vi "Make a Token.vi"() -> ()   [LabVIEW 2021]
uses:
  <vilib>/Utility/sysdir.llb/System Directory Type.ctl
  <vilib>/LabVIEW Icon API/API_User Layer Data.ctl
  <vilib>/Utility/miscctls.llb/LVPoint32TypeDef.ctl
  <vilib>/picture/picture.llb/imagedata.ctl
  <vilib>/Utility/miscctls.llb/LVPositionTypeDef.ctl
  <vilib>/LabVIEW Icon API/lv_icon/Classes/Icon/Icon.lvclass
  Material-Scheme/Material-Scheme.lvclass
  <vilib>/LabVIEW Icon API/LabVIEW Icon API.lvlib
panel:
  in  "New Color":u32(colorbox)=5263440
  in  "VI with Control":path=path "C:/Development/Open Source/tsc-material-theme/other-buttons/source/palette/token--image.vi"
  out "appended path":path[](array[path])
  in  "File Path":path[](array[path])
  out "error out":errorcluster
  in  "error in":errorcluster
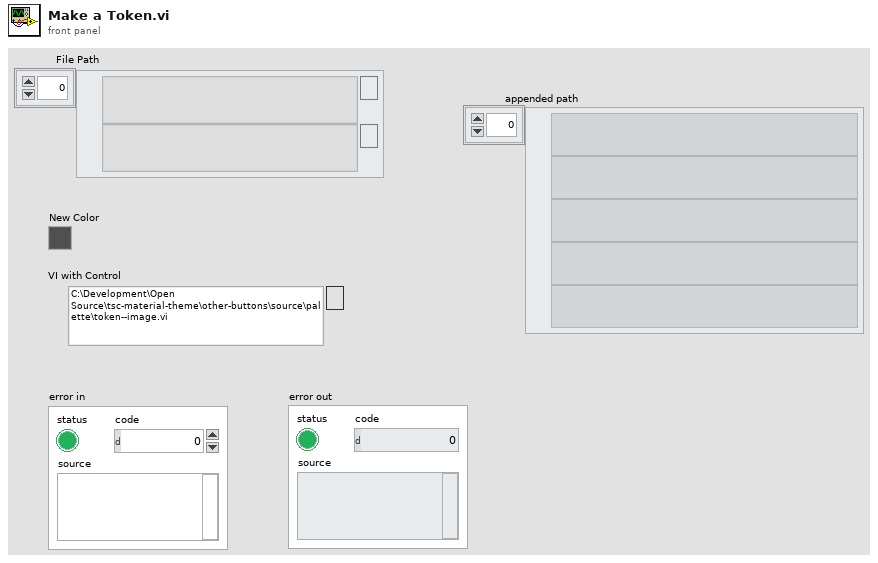
[diagram p1: front panel]
types:
  T1 = typedef "System Directory Type.ctl" = i32
  T2 = typedef "LVPoint32TypeDef.ctl" = cluster{"Horizontal":i32, "Vertical":i32}
  T3 = typedef "LabVIEW Icon API.lvlib/API_User Layer Data.ctl" = cluster{"Layer name":string, "Origin":T2, "Icon image data":T4}
  T4 = typedef "imagedata.ctl" = cluster{"image type":i32, "image depth":i32, "image":u8[], "mask":u8[], "colors":u32[], "Rectangle":cluster{"left":i16, "top":i16, "right":i16, "bottom":i16}}
  T5 = typedef "LVPositionTypeDef.ctl" = cluster{"Left":i32, "Top":i32}
  T6 = enum32{"invalid VI type", "Standard VI", "Control VI", "Global VI", "Polymorphic VI", "Configuration VI", "SubSystem", "Facade VI", "Method VI", "Statechart Diagram VI"}
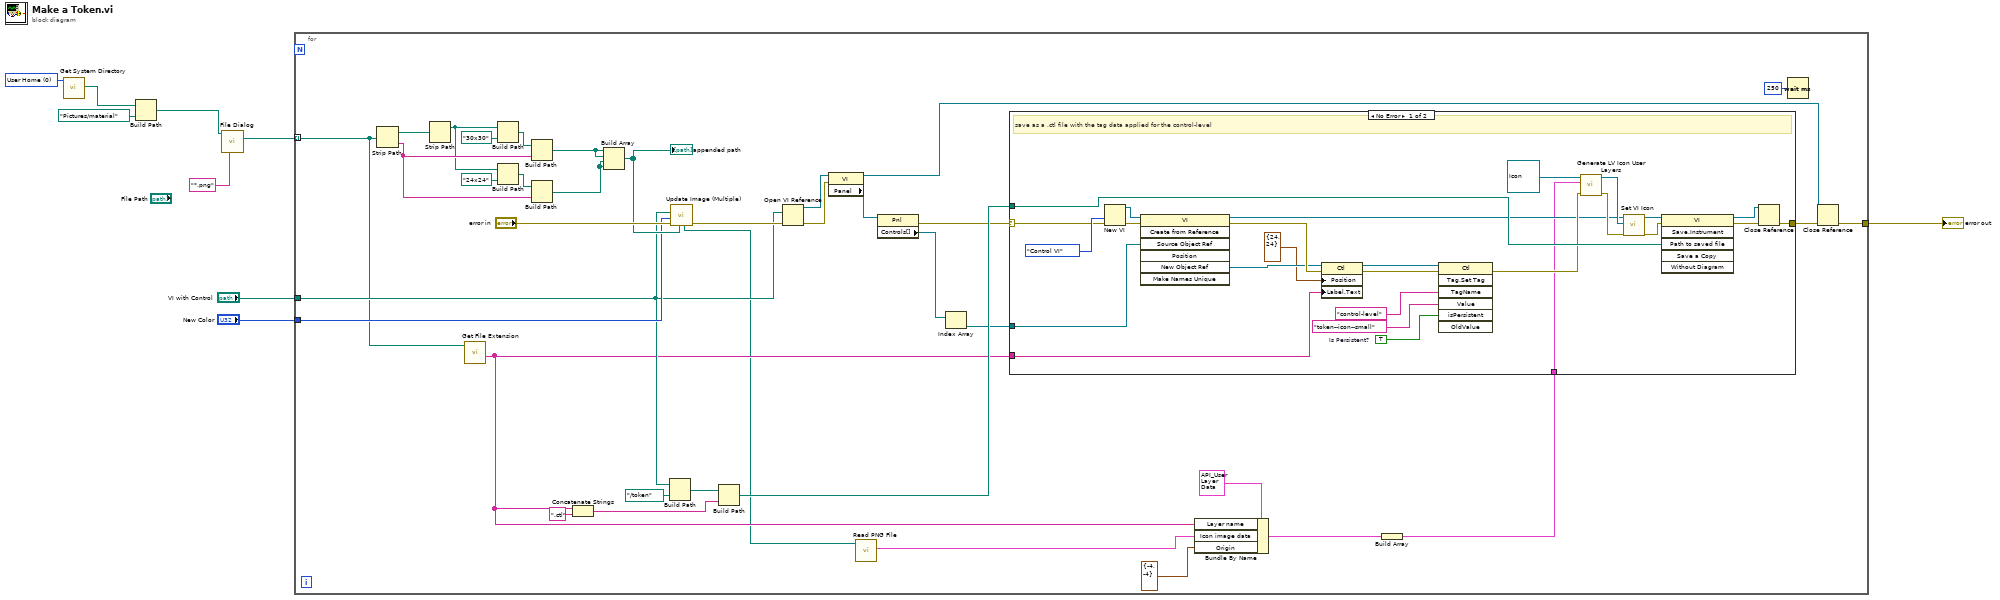
[diagram p0: block diagram]
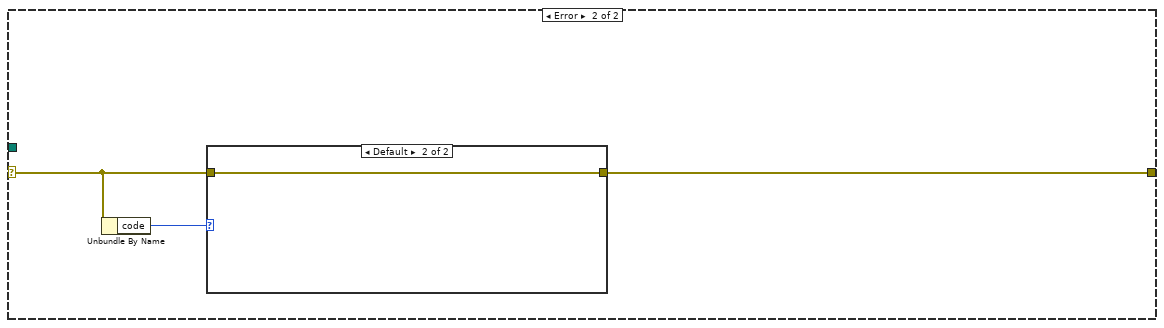
[diagram p2: hidden frame]
diagram:
  w4 = T1 0 items=["User Home"=0, "User Desktop"=1, "User Documents"=2, "User Application Data"=3, "User Preferences"=4, "User Temporary"=5, "Public Documents"=6, "Public Application Data"=7, "Public Preferences"=8, "Public Cache"=13, "System Core Libraries"=9, "System Installed Libraries"=10, "Application Files"=11, "Boot Volume Root"=12] ("system directory type")
  n1 = call <vilib>:"Get System Directory.vi"("system directory type"=w4) -> ("system directory"=w3:path)  [unwired: 10 in]
  n2 = Build Path(base path=w3, name or relative path=path "Pictures/material") -> (appended path=w1:path)
  n3 = call "File Dialog"("start path"=w1, "pattern (all files)"="*.png") -> ("selected paths"=w6:path[])  [unwired: 10 in, 3 out]
  n4 = for {
    tunnel: "New Color" -> [w35]
    tunnel: w6 -> [w17] mode=indexing
    tunnel: [w20] -> w8
    tunnel: "VI with Control" -> [w27]
    n5 = Strip Path(path=w17) -> (stripped path=w45:path, name=w39:string)
    n6 = Strip Path(path=w45) -> (stripped path=w38:path)  [unwired: 1 out]
    n7 = call <vilib>:"Get File Extension.vi"("file"=w17) -> ("filename without extension"=w13:string)  [unwired: 6 in, 4 out]
    n8 = Build Path(base path=w38, name or relative path=path "30x30") -> (appended path=w43:path)
    n9 = Build Path(base path=w38, name or relative path=path "24x24") -> (appended path=w42:path)
    n10 = Build Path(base path=w43, name or relative path=w39) -> (appended path=w40:path)
    n11 = Build Path(base path=w42, name or relative path=w39) -> (appended path=w37:path)
    n12 = Concatenate Strings(w13, ".ctl" ("string")) -> (w31:string)
    n13 = Build Array(w40, w40, w37, w37) -> (w36:path[])
    "appended path" <- w36
    n14 = Build Path(base path=w27, name or relative path=path "../token") -> (appended path=w32:path)
    n15 = call "Update Image (Multiple).vi"("Replace Image"=w36, "error in"="error in", "New Color"=w35, "New Control"=w27) -> ("error out"=w29:errorcluster, "image"=w12:path)  [unwired: 5 in, 1 out]
    n16 = Build Path(base path=w32, name or relative path=w31) -> (appended path=w30:path)
    n17 = Open VI Reference(vi path=w27, error in (no error)=w29) -> (vi reference=w24:refnum<vi>, error out=w23:errorcluster)  [unwired: 4 in]
    n18 = property class="VI"(reference=w24, error in=w23) -> (reference out=w19:refnum<vi>, "Panel"=w26:refnum<vi>)  [unwired: 1 out]
    n19 = call <vilib>:"Read PNG File.vi"("path to PNG file"=w12) -> ("image data"=w11:T4)  [unwired: 8 in, 2 out]
    n20 = property class="Pnl"(reference=w26) -> (error out=w22:errorcluster, "Controls[]"=w25:refnum<vi>[])  [unwired: 1 in, 1 out]
    n21 = Index Array(array=w25) -> (element=w21:refnum<vi>)  [unwired: 1 in]
    n22 = Bundle By Name(cluster=T3 {"Layer name"="", "Origin"={"Horizontal"=0, "Vertical"=0}, "Icon image data"={"image type"=0, "image depth"=0, "image"=[], "mask"=[], "colors"=[], "Rectangle"={"left"=0, "top"=0, "right"=0, "bottom"=0}}} ("User layer"), "Layer name"=w13, "Icon image data"=w11, "Origin"=T2 {"Horizontal"=-4, "Vertical"=-4}) -> (w15:T3)
    n23 = Build Array(w15) -> (w16:T3[])
    n24 = case shown="No Error" w22 {
      selector: w22 -> [w65 w74]
      tunnel: [w67 w73] -> w28
      tunnel: w30 -> [w64 _]
      tunnel: w21 -> [w57 _]
      tunnel: w13 -> [w55 _]
      tunnel: w16 -> [w47 _]
      frame No Error {
        w60 = TRUE  # Is Persistent?
        # "save as a .ctl file with the tag data applied for the control-level"
        n25 = New VI(8:w65, 9:T6."Control VI" ("vi type (standard vi)")) -> (0:w71:errorcluster, 3:w70:refnum<vi>)  [unwired: 5 in]
        n26 = invoke class="VI" method="Create from Reference"(reference=w70, error in=w71, "Source Object Ref"=w57) -> (reference out=w49:refnum<vi>, error out=w69:errorcluster, "New Object Ref"=w63:refnum<vi>)  [unwired: 4 in, 4 out]
        n27 = property class="Ctl"(reference=w63, error in=w69, "Position"=T5 {"Left"=24, "Top"=24}, "Label.Text"=w55) -> (reference out=w58:refnum<vi>, error out=w59:errorcluster)
        n28 = invoke class="Ctl" method="Tag.Set Tag"(reference=w58, error in=w59, "TagName"="control-level" ("Tag Name"), "Value"="token--icon--small" ("Tag Name"), "isPersistent"=w60) -> (error out=w52:errorcluster)  [unwired: 2 in, 6 out]
        n29 = call <vilib>:"Generate LV Icon User Layers.vi"("error in (no error)"=w52, "User layers"=w47, "Icon in"=refnum<class "Icon.lvclass"> refnum ("Icon.lvclass in")) -> ("error out"=w51:errorcluster, "Icon out"=w54:refnum<class "Icon.lvclass">)  [unwired: 7 in]
        n30 = call <vilib>:"Set VI Icon.vi"("error in (no error)"=w51, "Icon"=w54, "VI Refnum in"=w49) -> ("error out"=w48:errorcluster, "VI Refnum out"=w50:refnum<vi>)  [unwired: 7 in]
        n31 = invoke class="VI" method="Save.Instrument"(reference=w50, error in=w48, "Path to saved file"=w64) -> (reference out=w66:refnum<vi>, error out=w68:errorcluster)  [unwired: 3 in, 4 out]
        n32 = Close Reference(reference=w66, error in (no error)=w68) -> (error out=w67:errorcluster)
      }
      frame Error {
        n33 = Unbundle By Name(w74) -> ("code"=w75:i32)
        n34 = case shown="Default" w75 {
          tunnel: w74 -> [_ w76]
          tunnel: [_ w76] -> w73
          frame 43 {
          }
          frame Default {
          }
        }
      }
    }
    n35 = Wait (ms)(milliseconds to wait=u32 250) -> ()  [unwired: 1 out]
    n36 = Close Reference(reference=w19, error in (no error)=w28) -> (error out=w20:errorcluster)
  }
  "error out" <- w8
